vi "op_biti_l1.vi"() -> ()   [LabVIEW 2009]
uses:
  <vilib>/Platform/portaccess.llb/Out Port8.vi
panel:
  in  "Knob":u8(knob)=3 scale=0.0..7.0
  out "Numeric":dbl=8.0
  out "Array":bool[](array[boolean])=[FALSE, FALSE, FALSE, FALSE, TRUE, FALSE, FALSE, FALSE]
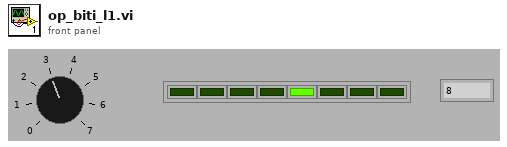
[diagram p1: front panel]
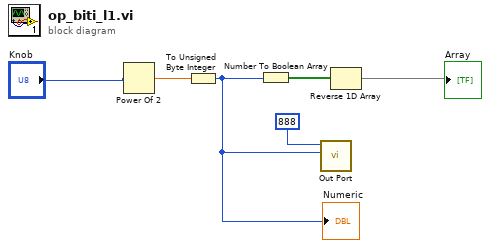
[diagram p0: block diagram]
diagram:
  n1 = Power Of 2(x="Knob") -> (2^x=w2:dbl)
  n2 = To Unsigned Byte Integer(number=w2) -> (unsigned 8bit integer=w1:u8)
  "Numeric" <- w1
  n3 = Number To Boolean Array(number=w1) -> (Boolean array=w4:bool[])
  n4 = call-poly <vilib>:"Out Port.vi"("write value"=w1, "address"=888) -> ()  [unwired: 7 in, 1 out]
  n5 = Reverse 1D Array(array=w4) -> (reversed array=→"Array":bool[])
